vi "SystemLink_Write_Number.vi"(9 "Numeric":dbl, 11 "SL_XControl":string(xcontrol)) -> ()   [LabVIEW 2020]
uses:
  SL_XControl.xctl
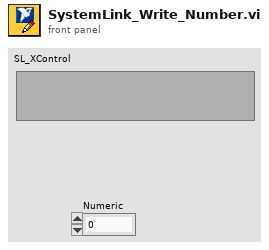
[diagram p1: front panel]
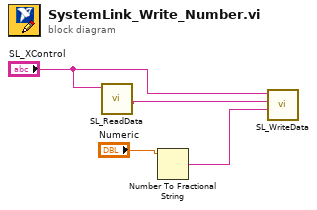
[diagram p0: block diagram]
diagram:
  n1 = call "SL_ReadData.vi"("Property"="SL_XControl") -> ("type"=w1:string)  [unwired: 9 in, 1 out]
  n2 = Number To Fractional String(number="Numeric") -> (F-format string=w3:string)  [unwired: 3 in]
  n3 = call "SL_WriteData.vi"("Data"=w3, "Type"=w1, "Path"="SL_XControl") -> ()  [unwired: 9 in]
